vi "FilterSRsStats(SubVI).vi"(7 "Filter Parameters":string[](array[string])=["Created in Error", "Declined to Purchase Support", "Expired", "Forum Resolved Customer", "RMA Approved for Return", "RMA Closed", "RMA In Progress", "RMA Open", "Status"], 8 "error in (no error)":errorcluster, 11 "Data Value Reference in":refnum<data-value>) -> (0 "error out":errorcluster, 3 "Data Value Reference out":refnum<data-value>, 6 "Filtered Out SRs":T1[](array[typedef]))   [LabVIEW 2017, in "DS_Lib.lvlib" / "SRReportParser.lvlib"]
uses:
  SRReportParser.lvlib
  Modules/Private Controls/Report Data Cluster.ctl
  Modules/Private Controls/Data Raw.ctl
  Modules/Data Operations.lvlib
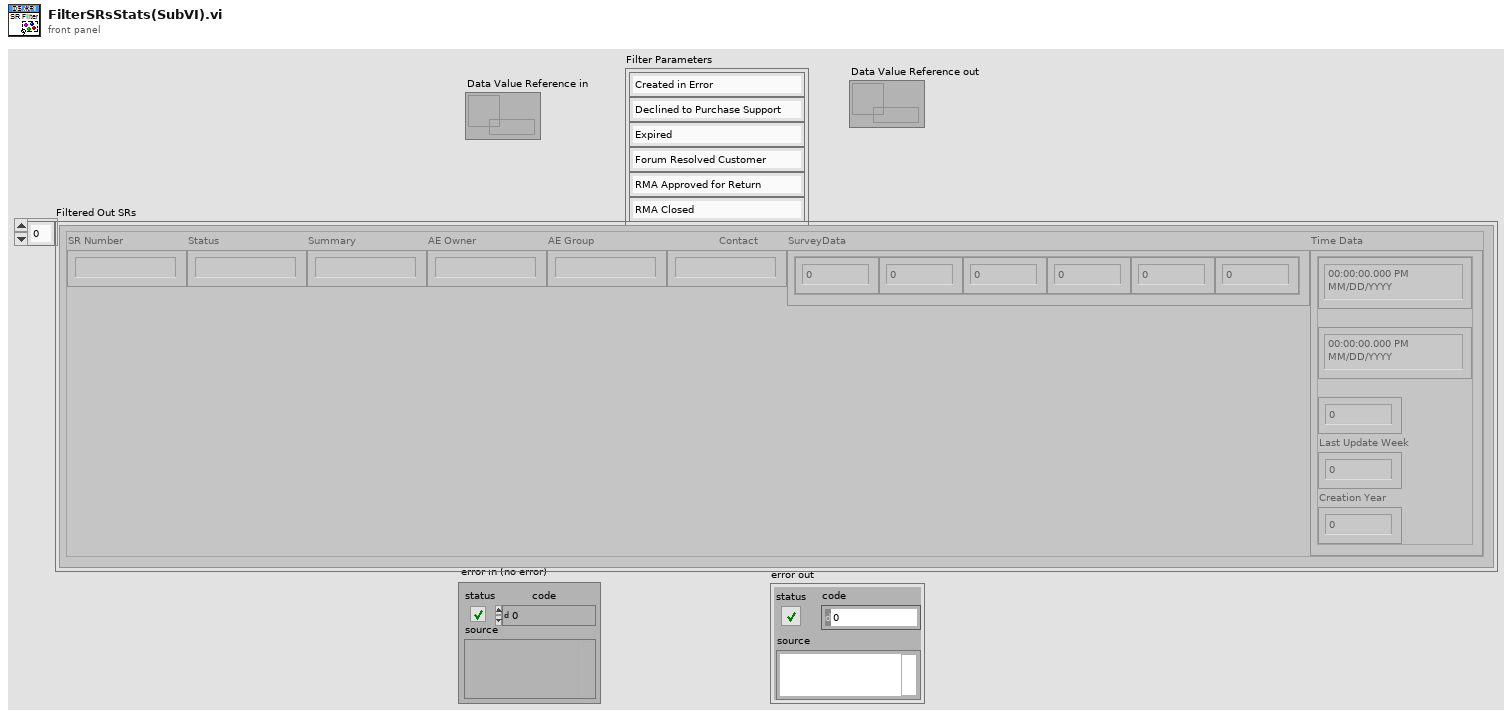
[diagram p1: front panel]
types:
  T1 = typedef "Data Operations.lvlib/Data Raw.ctl" = cluster{"SR Number":string, "Status":string, "Summary":string, "AE Owner":string, "AE Group":string, "Contact":string, "SurveyData":cluster{"Resolution Time":dbl, "Total Satisfaction":dbl, "Response Time":dbl, "Courtesy":dbl, "Problem Solved":dbl, "Level of effort":dbl}, "Time Data":cluster{"Last Update Date":timestamp, "Creation Date":timestamp, "Creation week":i16, "Last Update Week":i16, "Creation Year":i16}}
  T2 = typedef "Data Operations.lvlib/Report Data Cluster.ctl" = cluster{"Headers":cluster{"Start Date":timestamp, "End Date":timestamp, "SR Status String":string[], "AE Owner String":string[]}, "Data":T1[]}
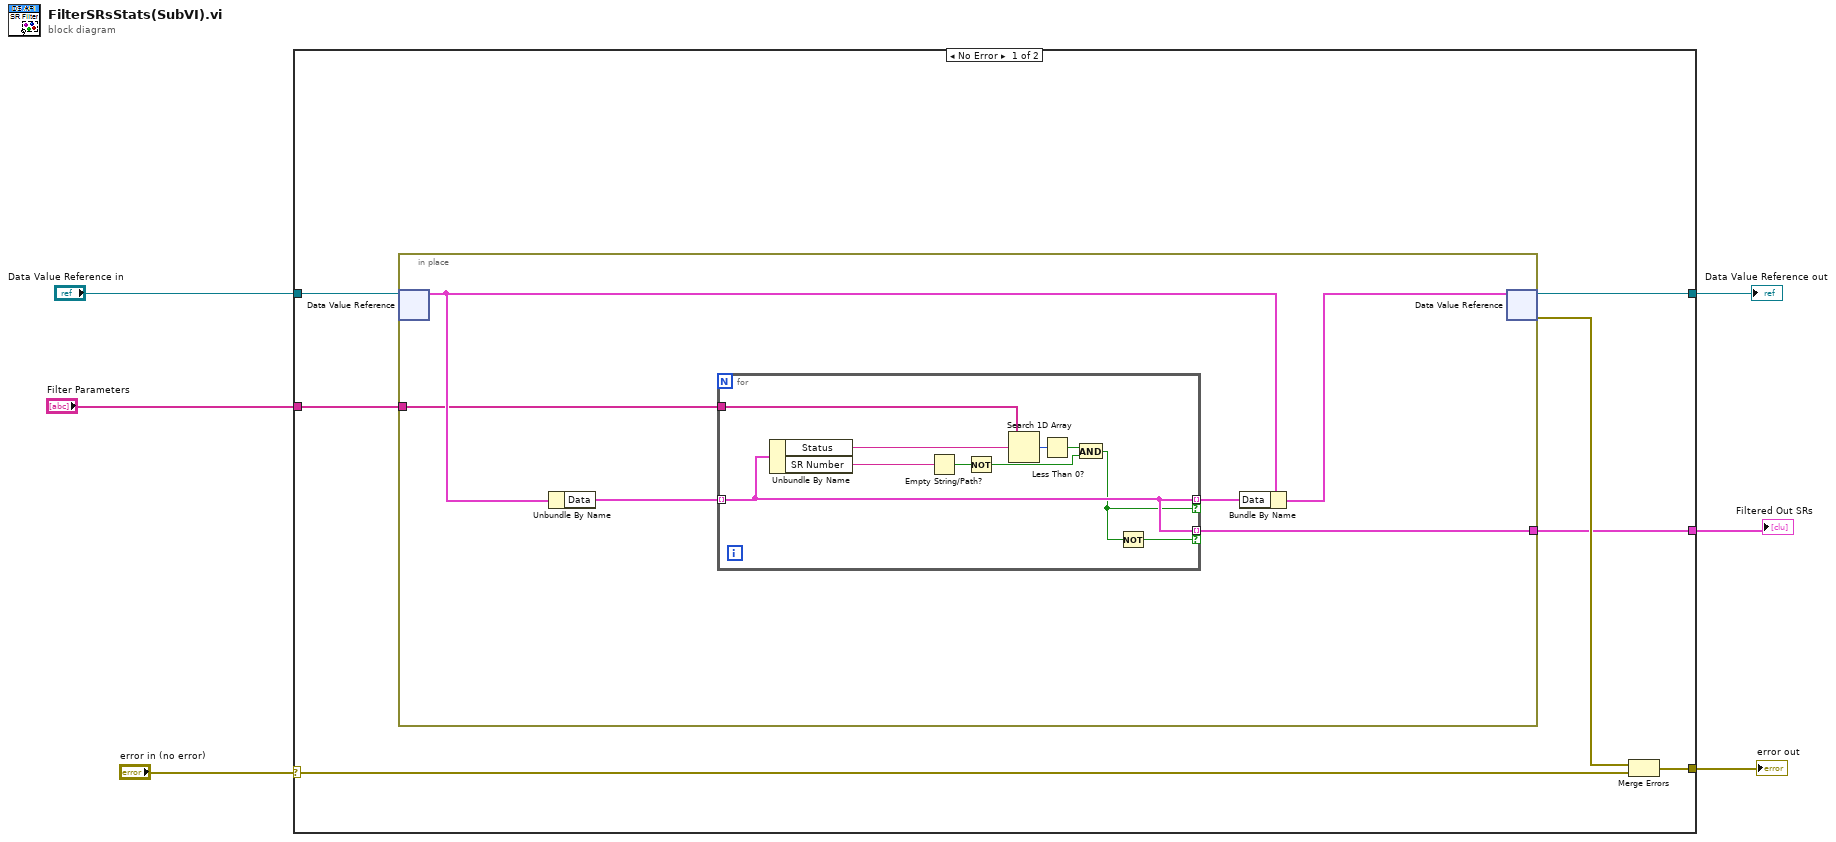
[diagram p0: block diagram]
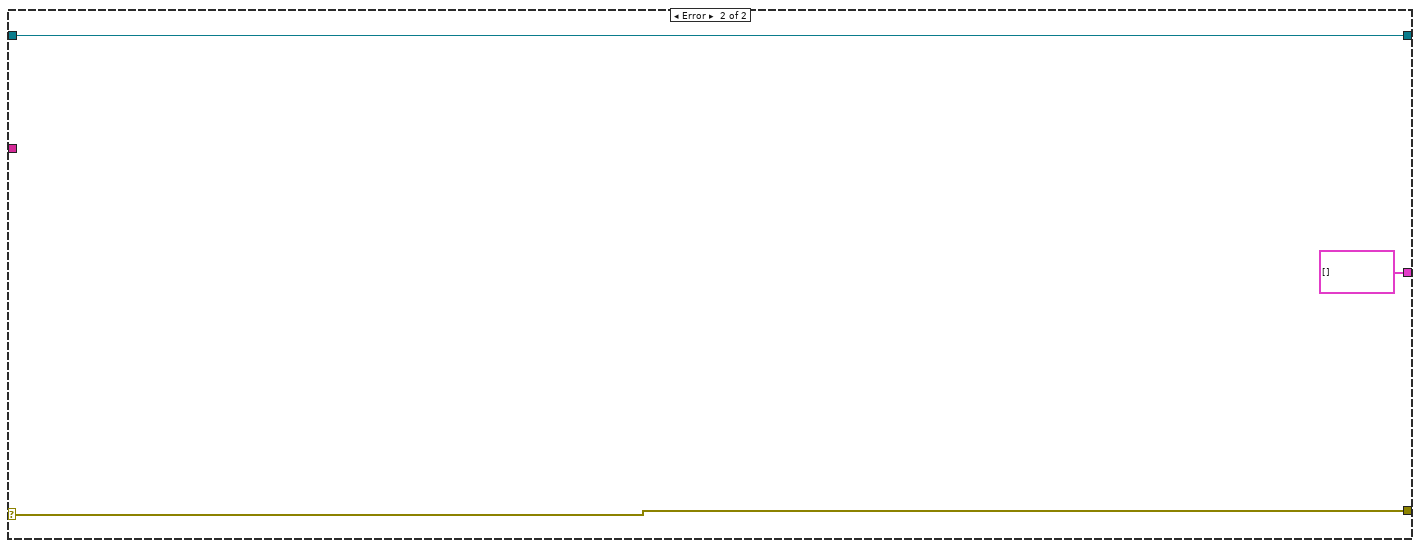
[diagram p2: hidden frame]
diagram:
  n1 = case shown="No Error" "error in (no error)" {
    selector: "error in (no error)" -> [w8 w32]
    tunnel: [w10 w32] -> w6
    tunnel: [w12 w31] -> w2
    tunnel: "Data Value Reference in" -> [w11 w31]
    tunnel: "Filter Parameters" -> [w13 _]
    tunnel: [w7 T1[] []] -> w1
    frame No Error {
      n2 = in-place {
        in-place-border: w13 -> [w17]
        in-place-border: [w14] -> w7
        n3 = in-place-dvr #1(w11) -> (w19:T2)  [unwired: 1 out]
        n4 = Unbundle By Name(w19) -> ("Data"=w16:T1[])
        n5 = for {
          tunnel: w16 -> [w27] mode=indexing
          tunnel: w17 -> [w29]
          tunnel: [w27] -> w15 mode=indexing if=w20
          tunnel: [w27] -> w14 mode=indexing if=w26
          n6 = Unbundle By Name(w27) -> ("Status"=w23:string, "SR Number"=w24:string)
          n7 = Empty String/Path?(string/path=w24) -> (empty?=w25:bool)
          n8 = Not(x=w25) -> (.not. x?=w21:bool)
          n9 = Search 1D Array(1D array=w29, element=w23) -> (index of element=w28:i32)  [unwired: 1 in]
          n10 = Less Than 0?(x=w28) -> (x < 0?=w22:bool)
          n11 = And(x=w22, y=w21) -> (x .and. y?=w20:bool)
          n12 = Not(x=w20) -> (.not. x?=w26:bool)
        }
        n13 = Bundle By Name(cluster=w19, "Data"=w15) -> (w18:T2)
        n14 = in-place-dvr #1(w18) -> (w12:refnum<data-value>, w9:errorcluster)
      }
      n15 = Merge Errors(w9, w8) -> (w10:errorcluster)
    }
    frame Error {
    }
  }
  "error out" <- w6
  "Data Value Reference out" <- w2
  "Filtered Out SRs" <- w1
